vi "oa_Check Channel Info [OPS] (N Channels).vi"(6 "channel info":T1[](array[typedef]) {"channel info"."pregain" format="%.2f"; "channel info"."weighting filter" items=["Linear", "A-weighting", "B-weighting", "C-weighting", "ITU-R 468-4", "Dolby", "CCITT", "C-message", "Wb", "Wc", "Wd", "We", "Wf", "Wh", "Wj", "Wk", "Wm", "AES17 20 kHz lowpass", "AES17 40 kHz lowpass", "AES17 20 kHz highpass", "AES17 40 kHz highpass"]; "channel info"."dB reference" format="%^.1e"; "channel info"."engineering units" items=["custom..."=0, "V"=1, "A"=21, "C"=30, "pC"=31, "s"=32, "-"=29, "Pa"=2, "N"=20, "g"=3, "m/s^2"=4, "m/s"=5, "m"=6, "mm/s"=12, "mm"=13, "micron/s"=14, "micron"=15, "in/s^2"=7, "in/s"=8, "in"=9, "mil/s"=10, "mil"=11, "rad/s^2"=16, "rad/s"=17, "rad"=18, "deg/s^2"=26, "deg/s"=27, "deg"=28, "RPM"=22, "cycle/s^2"=23, "Hz"=24, "cycle"=25, "strain"=19]; "channel info"."sensor sensitivity" format="%#_5f"}, 8 "error in (no error)":errorcluster, 11 "resampled signal":cluster{"r0":dbl, "dr":dbl, "Y":dbl[]}[](array[cluster]) {"r0" format="%.2p"; "dr" format="%.2p"; "Y" format="%.2f"}) -> (0 "error out":errorcluster, 1 "parameter changed":bool, 3 "resampled signal out":cluster{"r0":dbl, "dr":dbl, "Y":dbl[]}[](array[cluster]))   [LabVIEW 2017, in "SoundVib_Resampling.lvlib"]
uses:
  <vilib>/addons/Sound and Vibration/Order Analysis/Resample Order Tracking/SoundVib_Resampling.lvlib
  <vilib>/addons/_NISVFA/_Shared subVIs/Controls/svc_Resampled Channel Info.ctl
  <vilib>/addons/_NISVFA/_Shared subVIs/Controls/svc_Channel Info.ctl
  <vilib>/addons/_NISVFA/_Shared subVIs/Controls/svc_Engineering Units Text Ring.ctl
  <vilib>/addons/_NISVFA/_Shared subVIs/Controls/svc_Weighting Filter Text Ring.ctl
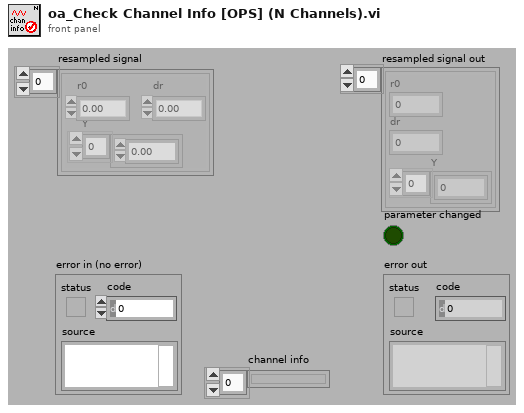
[diagram p1: front panel]
types:
  T1 = typedef "svc_Resampled Channel Info.ctl" = cluster{"channel name":string, "description":string, " channel info":T2}
  T2 = typedef "svc_Channel Info.ctl" = cluster{"sensor sensitivity":dbl, "engineering units":T3, "dB reference":dbl, "custom label":string, "weighting filter":T4, "pregain":dbl}
  T3 = typedef "svc_Engineering Units Text Ring.ctl" = u16
  T4 = typedef "svc_Weighting Filter Text Ring.ctl" = u16
  T5 = cluster{"ignore dt's equal":bool, "ignore array lengths equal":bool, "ignore # channels":bool}
  T6 = cluster{"ignore dt":bool, "ignore t0 continuity":bool, "ignore array length":bool, "ignore channel info":bool, "ignore channel name":bool}
  T7 = cluster{"r0":dbl, "dr":dbl, "even angle signal":dbl[]}[]
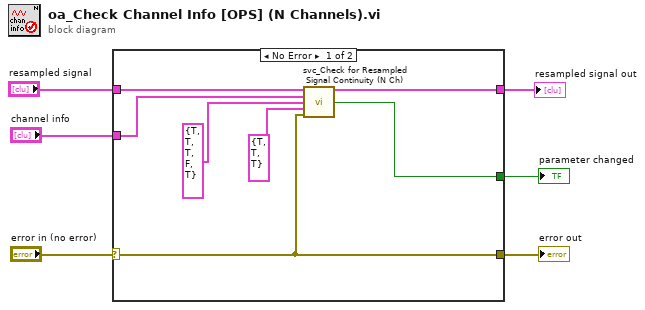
[diagram p0: block diagram]
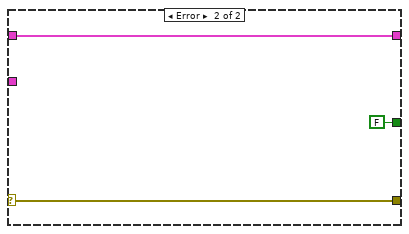
[diagram p2: hidden frame]
diagram:
  n1 = case shown="No Error" "error in (no error)" {
    selector: "error in (no error)" -> [w7 w16]
    tunnel: [w7 w16] -> w5
    tunnel: "channel info" -> [w12 _]
    tunnel: [w8 FALSE] -> w3
    tunnel: "resampled signal" -> [w13 w14]
    tunnel: [w11 w14] -> w1
    frame No Error {
      n2 = call <vilib>:"svc_Check for Resampled Signal Continuity (N Ch).vi"("even angle signals"=w13, "even angle channel info"=w12, "parameter controls"=T6 {"ignore dt"=TRUE, "ignore t0 continuity"=TRUE, "ignore array length"=TRUE, "ignore channel info"=FALSE, "ignore channel name"=TRUE}, "multichannel parameter controls"=T5 {"ignore dt's equal"=TRUE, "ignore array lengths equal"=TRUE, "ignore # channels"=TRUE}, "error in (no error)"=w7) -> ("dup even angle signals"=w11:T7, "waveform parameter changed"=w8:bool)  [unwired: 4 in, 5 out]
    }
    frame Error {
    }
  }
  "error out" <- w5
  "resampled signal out" <- w1
  "parameter changed" <- w3
